vi "coag dose.vi"(9 "DOM coag demand (mg/L)":dbl, 10 "raw water turbidity (NTU)":dbl, 11 "Coagulant":T1={"flocculator volume (L)"=66.81, "clarifier volume (L)"=1336.0, "dose updates per response delay"=10, "target clarified turbidity (NTU)"=0.6, "Coagulant mode"=enum."manual", "Coag dose [mg/L]"=5.5, "pump mL/rev"=0.255, "clarifier flow [L/s]"=0.5, "min Coag dose [mg/L]"=0.0, "max Coag dose [mg/L]"=0.0, "Steps"=3, "HRT response delay"=1, "kpf"=1.0, "DOM coag demand [mg/L]"=0.0, "min DOM coag demand [mg/L]"=0.0, "max DOM coag demand [mg/L]"=0.0} {"max DOM coag demand [mg/L]" min=0.0 max=20.0 step=0.1; "min DOM coag demand [mg/L]" min=0.0 max=10.0 step=0.1; "DOM coag demand [mg/L]" min=0.0 max=20.0 step=0.1; "HRT response delay" min=1 max=10 step=1; "Steps" min=3 step=1; "clarifier flow [L/s]" min=0.0001 max=1.0 step=0.0001; "target clarified turbidity (NTU)" min=0.1 max=5.0 step=0.01; "dose updates per response delay" min=1 max=100 step=1}) -> (3 "coag dose (mg/L)":dbl)   [LabVIEW 2019]
uses:
  coag.ctl
  model type.ctl
panel:
  # "ramp controls"
  # "min"
  # "max"
  # "min"
  # "max"
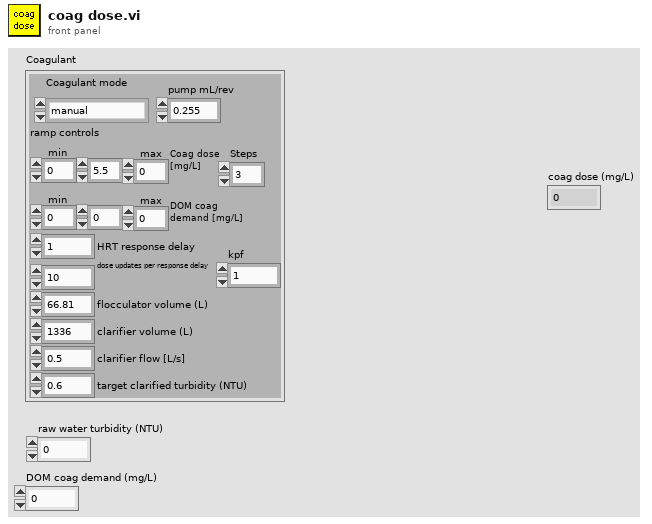
[diagram p1: front panel]
types:
  T1 = typedef "coag.ctl" = cluster{"flocculator volume (L)":dbl, "clarifier volume (L)":dbl, "dose updates per response delay":u16, "target clarified turbidity (NTU)":dbl, "Coagulant mode":T2, "Coag dose [mg/L]":dbl, "pump mL/rev":dbl, "clarifier flow [L/s]":dbl, "min Coag dose [mg/L]":dbl, "max Coag dose [mg/L]":dbl, "Steps":u16, "HRT response delay":u32, "kpf":dbl, "DOM coag demand [mg/L]":dbl, "min DOM coag demand [mg/L]":dbl, "max DOM coag demand [mg/L]":dbl}
  T2 = typedef "model type.ctl" = enum16{"manual", "ramp", "simple corrector"}
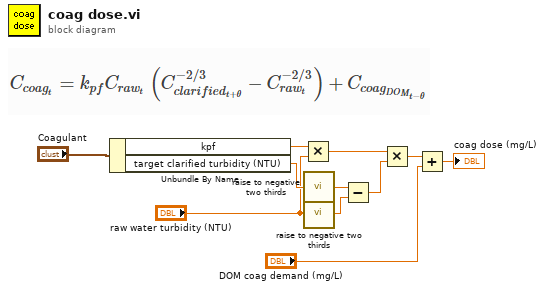
[diagram p0: block diagram]
diagram:
  n1 = Unbundle By Name("Coagulant") -> ("kpf"=w5:dbl, "target clarified turbidity (NTU)"=w6:dbl)
  n2 = Multiply(x=w5, y="raw water turbidity (NTU)") -> (x*y=w7:dbl)
  n3 = call "raise to negative two thirds.vi"("Numeric in"=w6) -> ("Numeric out"=w10:dbl)  [unwired: 4 in]
  n4 = call "raise to negative two thirds.vi"("Numeric in"="raw water turbidity (NTU)") -> ("Numeric out"=w9:dbl)  [unwired: 4 in]
  n5 = Subtract(x=w10, y=w9) -> (x-y=w8:dbl)
  n6 = Multiply(x=w7, y=w8) -> (x*y=w11:dbl)
  n7 = Add(x=w11, y="DOM coag demand (mg/L)") -> (x+y=→"coag dose (mg/L)":dbl)
